vi "Write Power Meter classes.vi"(10 "Power Meter classes":refnum<class "Power Meter.lvclass">[](array[class]), 11 "RF Power in":refnum<class "RF Power.lvclass">) -> (3 "RF Power out":refnum<class "RF Power.lvclass">)   [LabVIEW 2020, in "RF Power.lvclass"]
uses:
  RF Power.lvclass
  Instruments/Power Meter/Power Meter.lvclass
  RF Power.lvclass/RF Power.ctl
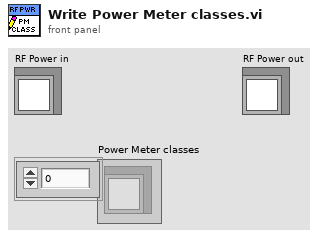
[diagram p1: front panel]
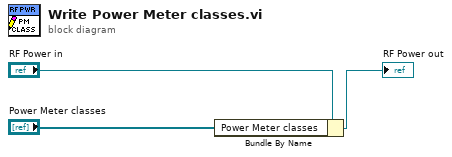
[diagram p0: block diagram]
diagram:
  n1 = Bundle By Name(cluster="RF Power in", "Power Meter classes"="Power Meter classes") -> (→"RF Power out":refnum<class "RF Power.lvclass">)
